vi "runscenario estimate time.vi"(6 "User":string, 8 "error in (no error)":errorcluster, 10 "Templates":T1[](array[typedef]), 11 "runs":T2[](array[typedef])) -> (0 "error out":errorcluster, 3 "estimate (secs)":i32)   [LabVIEW 2011]
uses:
  _cgi-lib/TDM_INDEX Record.ctl
  server/database/Templates/Template Record.ctl
  server/DIAdem/Datasheet/Datasheet Generator Settings.ctl
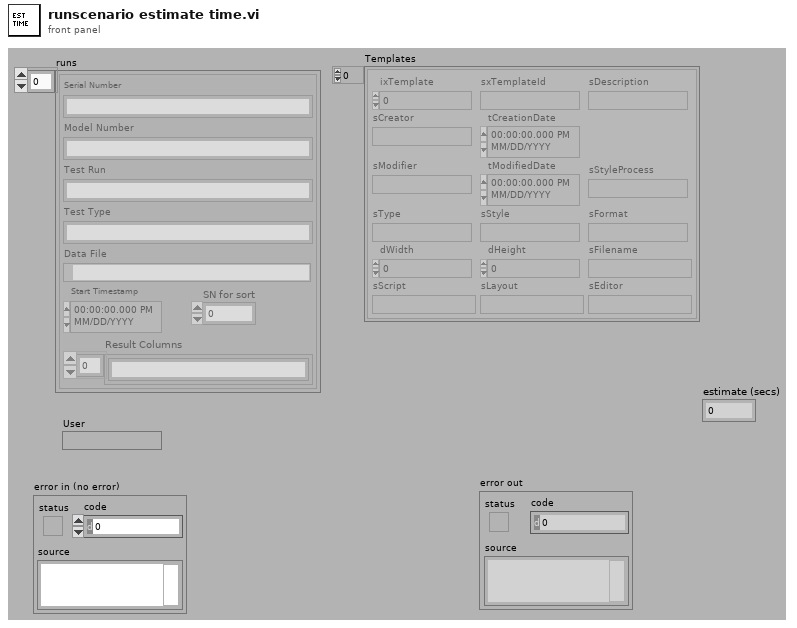
[diagram p1: front panel]
types:
  T1 = typedef "Template Record.ctl" = cluster{"ixTemplate":i32, "sxTemplateId":string, "sDescription":string, "sCreator":string, "tCreationDate":timestamp, "sModifier":string, "tModifiedDate":timestamp, "sType":string, "sStyle":string, "sFormat":string, "dWidth":dbl, "dHeight":dbl, "sFilename":string, "sScript":string, "sLayout":string, "sEditor":string, "sStyleProcess":string}
  T2 = typedef "TDM_INDEX Record.ctl" = cluster{"Model Number":string, "SN for sort":i32, "Test Type":string, "Test Run":string, "Serial Number":string, "Start Timestamp":timestamp, "Data File":path, "Result Columns":string[]}
  T3 = typedef "DATASHEET Generator Settings.ctl" = cluster{"Wait? (t)":bool, "ClientPrint? (f)":bool, "Client (\"\")":string, "joinPDF":bool, "Sort Method":enum16{"Item", "Template", "No Sort"}, "Export Row (-1=all)":i32, "Preview":bool, "Estimate Time":bool, "username":string, "jobid":string}
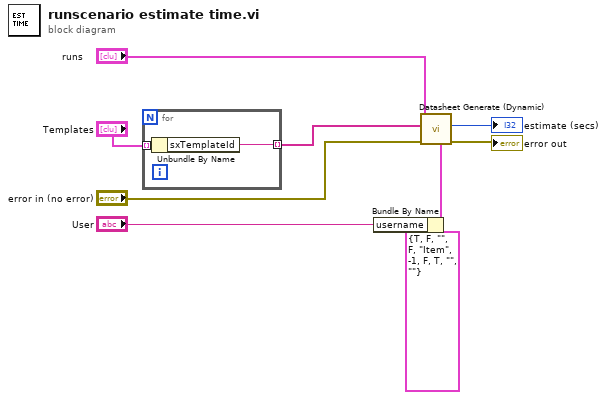
[diagram p0: block diagram]
diagram:
  n1 = for {
    tunnel: "Templates" -> [w11] mode=indexing
    tunnel: [w10] -> w8 mode=indexing
    n2 = Unbundle By Name(w11) -> ("sxTemplateId"=w10:string)
  }
  n3 = Bundle By Name(cluster=T3 {"Wait? (t)"=TRUE, "ClientPrint? (f)"=FALSE, "Client (\"\")"="", "joinPDF"=FALSE, "Sort Method"=enum."Item", "Export Row (-1=all)"=-1, "Preview"=FALSE, "Estimate Time"=TRUE, "username"="", "jobid"=""} ("Generator Settings"), "username"="User") -> (w6:T3)
  n4 = call "Datasheet Generate (Dynamic).vi"("Generator Settings"=w6, "error in (no error)"="error in (no error)", "Templates"=w8, "Items"="runs") -> ("error out"=→"error out":errorcluster, "Actual (sec)"=→"estimate (secs)":i32)  [unwired: 5 in, 1 out]
